vi "Temperature alarm.vi"() -> ()   [LabVIEW 2018]
uses:
  <vilib>/Utility/file.llb/Read Delimited Spreadsheet (I64).vi
panel:
  in  "Maximum Temperature":dbl
  out "Alarm":bool
  out "Waveform Chart":T1(graph)
  in  "file path (dialog if empty)":path
  # "Temperature Warning"
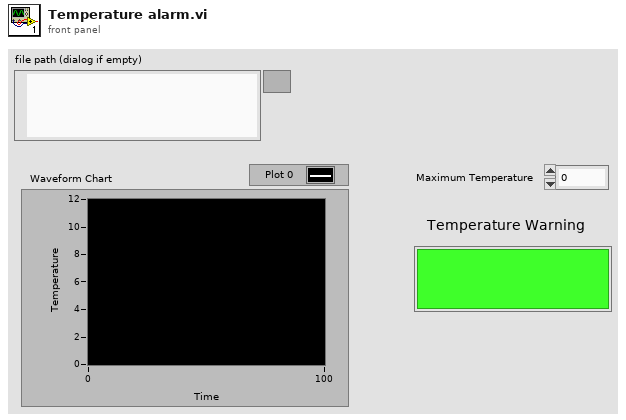
[diagram p1: front panel]
types:
  T1 = cluster{"Numeric":i64, "Maximum Temperature":dbl}
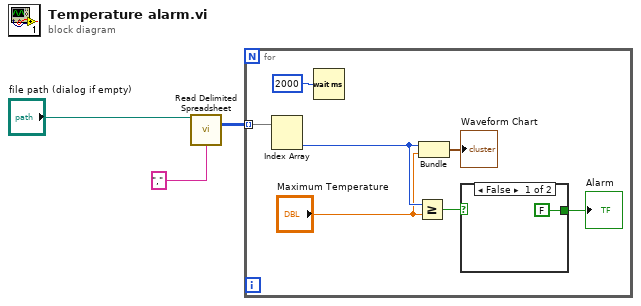
[diagram p0: block diagram]
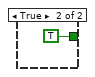
[diagram p2: hidden frame]
diagram:
  n1 = call-poly <vilib>:"Read Delimited Spreadsheet.vi"("file path (dialog if empty)"="file path (dialog if empty)", "delimiter (\\t)"="," ("delimiter (\\t)")) -> ("all rows"=w3:i64[][])  [unwired: 8 in, 5 out]
  n2 = for {
    tunnel: w3 -> [w9] mode=indexing
    n3 = Index Array(array=w9) -> (element #2=w6:i64)  [unwired: 2 in, 1 out]
    n4 = Wait (ms)(milliseconds to wait=u32 2000) -> ()  [unwired: 1 out]
    n5 = Greater Or Equal?(x=w6, y="Maximum Temperature") -> (x >= y?=w8:bool)
    n6 = Bundle("Numeric"=w6, "Maximum Temperature"="Maximum Temperature") -> (→"Waveform Chart":T1)  [unwired: 1 in]
    n7 = case shown="False" w8 {
      tunnel: [FALSE TRUE ("Boolean")] -> w7
      frame False {
      }
      frame True {
      }
    }
    "Alarm" <- w7
  }
